vi "Set sel exp.vi"(8 "error in (no error)":errorcluster, 10 "Experiment":refnum<class "Experiment.lvclass">, 11 "Control-Client in":refnum<class "Control-Client.lvclass">) -> (0 "error out":errorcluster, 3 "Control-Client out":refnum<class "Control-Client.lvclass">)   [LabVIEW 2019, in "Control-Client.lvclass"]
uses:
  Control-Client.lvclass
  Experiments/Experiment.lvclass
  Control-Client.lvclass/Control-Client.ctl
  methods/Read Group #.vi
  Experiments/Experiments_group.lvclass
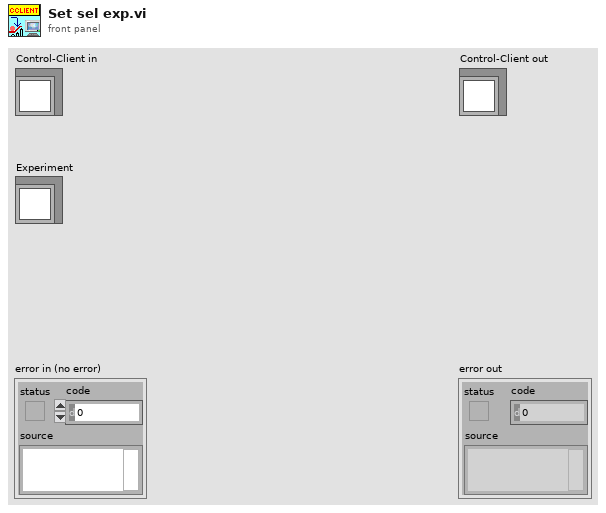
[diagram p1: front panel]
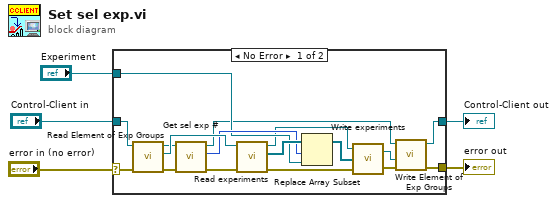
[diagram p0: block diagram]
diagram:
  n1 = case shown="No Error" "error in (no error)" {
    selector: "error in (no error)" -> [w22 w24]
    tunnel: [w16 w24] -> w4
    tunnel: [w15 w23] -> w2
    tunnel: "Control-Client in" -> [w17 w23]
    tunnel: "Experiment" -> [w18 _]
    frame No Error {
      n2 = call "Read Element of Exp Groups.vi"("error in (no error)"=w22, "Control-Client in"=w17) -> ("error out"=w7:errorcluster, "Experiments_group.lvclass"=w21:refnum<class "Experiments_group.lvclass">, "Control-Client out"=w9:refnum<class "Control-Client.lvclass">)  [unwired: 7 in]
      n3 = call "Get sel exp #.vi"("error in (no error)"=w7, "Control-Client in"=w9) -> ("error out"=w8:errorcluster, "Exp sel #"=w19:i32, "Control-Client out"=w10:refnum<class "Control-Client.lvclass">)  [unwired: 7 in]
      n4 = call "Read experiments.vi"("error in (no error)"=w8, "Experiments_group.lvclass in"=w21) -> ("error out"=w12:errorcluster, "Experiments"=w20:refnum<class "Experiment.lvclass">[], "Experiments_group.lvclass out"=w14:refnum<class "Experiments_group.lvclass">)  [unwired: 6 in]
      n5 = Replace Array Subset(array=w20, new element=w18, index=w19) -> (w13:refnum<class "Experiment.lvclass">[])
      n6 = call-dynamic "Write experiments.vi"("error in (no error)"=w12, "Experiments"=w13, "Experiments_group.lvclass in"=w14) -> ("error out"=w6:errorcluster, "Experiments_group.lvclass out"=w11:refnum<class "Experiments_group.lvclass">)
      n7 = call "Write Element of Exp Groups.vi"("error in (no error)"=w6, "Experiments_group.lvclass"=w11, "Control-Client in"=w10) -> ("error out"=w16:errorcluster, "Control-Client out"=w15:refnum<class "Control-Client.lvclass">)  [unwired: 7 in]
    }
    frame Error {
    }
  }
  "error out" <- w4
  "Control-Client out" <- w2
